vi "WinBuilder.vi"(6 "Wvfrm_ref":T1={"t0"=timestamp(0 s since 1904-01-01), "dt"=1.0, "attributes"=variant, "Y_ref"=refnum} {"dt" format="%0.6f"; "t0" format="%<%X\n%x>T"}, 8 "error in (no error)":errorcluster, 9 "AnalysisTime":dbl, 10 "clAnalysisConfig":T3={"F0"=60, "SettlingTime"=7.0, "AnalysisCycles"=20.0, "SampleRate"=4800.0, "NumChannels"=6, "TsOffset"=enum."start"}, 11 "Window":T2 {"T0" format="%.6f"; "Timestamp" format="%.6f"}) -> (0 "error out":errorcluster, 1 "Continue":bool, 2 "Valid":bool, 3 "Window":T2 {"T0" format="%.6f"; "Timestamp" format="%.6f"}, 4 "Wvfrm_ref":T1={"t0"=timestamp(0 s since 1904-01-01), "dt"=1.0, "attributes"=variant, "Y_ref"=refnum} {"dt" format="%0.6f"; "t0" format="%<%X\n%x>T"})   [LabVIEW 2018, in "AnalysisPlugins.lvlib" / "FitterBase.lvclass"]
uses:
  FitterBase.lvclass
  AnalysisPluginBaseClass/Typedefs/clWindowData.ctl
  Typedefs/clAnalysisConfig.ctl
  Typedefs/Wvfrm_ref.ctl
  Digitizer/DigitizerPlugins/DigitizerBaseClass/Typedefs/WfrmAttributes.ctl
  Digitizer/DigitizerPlugins/DigitizerBaseClass/DigitizerBase.lvclass
  AnalysisPluginBaseClass/AnalysisPluginsBase.lvclass
panel:
  out "AnalysisTime":timestamp
  out "SampleStartTime":timestamp
  out "TimestampNeeded":timestamp
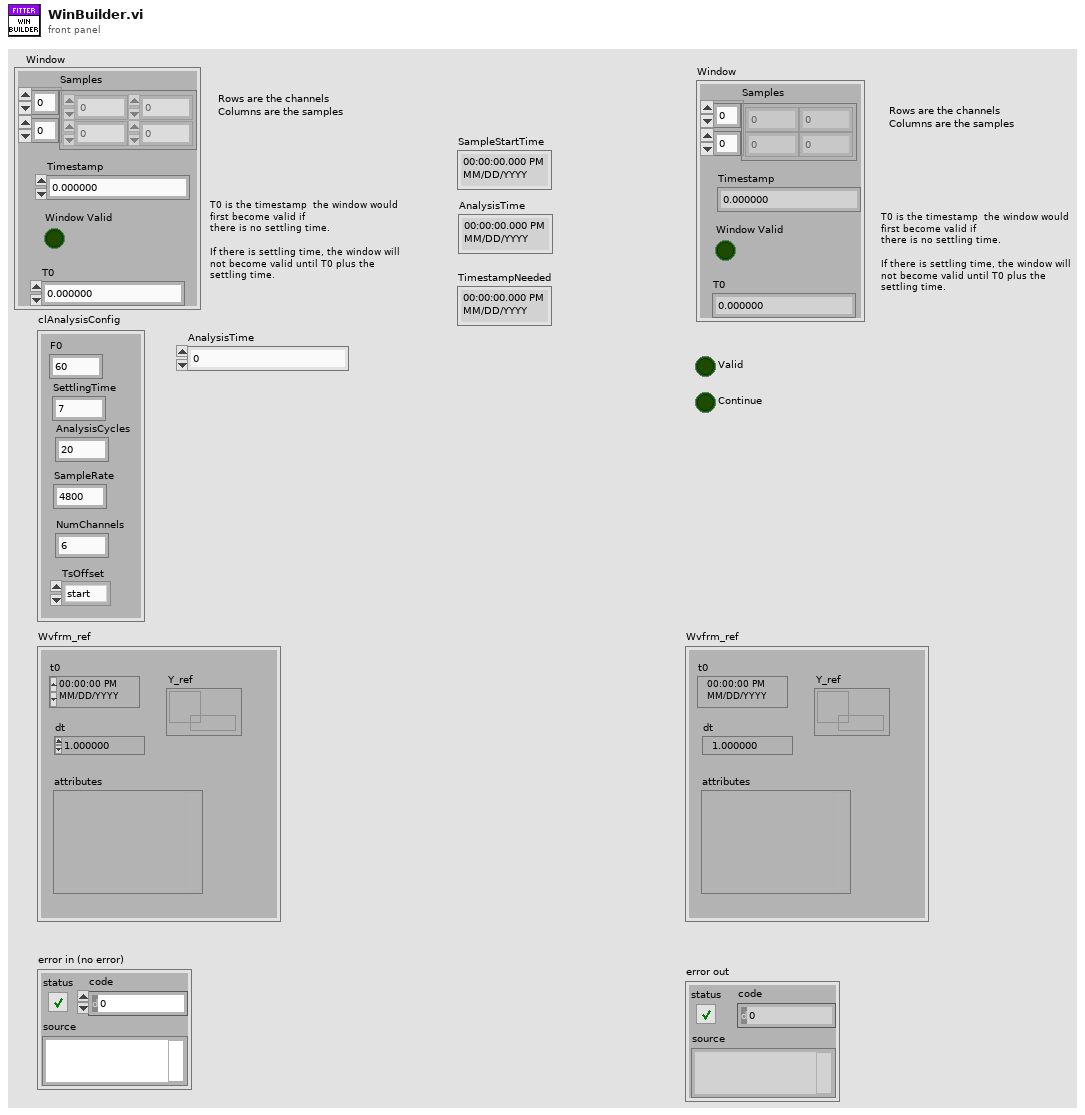
[diagram p1: front panel]
types:
  T1 = typedef "AnalysisPlugins.lvlib/FitterBase.lvclass/Wvfrm_ref.ctl" = cluster{"t0":timestamp, "dt":dbl, "attributes":variant, "Y_ref":refnum<data-value>}
  T2 = typedef "AnalysisPlugins.lvlib/AnalysisPluginsBase.lvclass/clWindowData.ctl" = cluster{"Timestamp":ext, "Samples":dbl[][], "Window Valid":bool, "T0":ext}
  T3 = typedef "AnalysisPlugins.lvlib/FitterBase.lvclass/clAnalysisConfig.ctl" = cluster{"F0":u32, "SettlingTime":dbl, "AnalysisCycles":dbl, "SampleRate":dbl, "NumChannels":u32, "TsOffset":enum16{"start", "middle", "end"}}
  T4 = typedef "DigitizerPlugins.lvlib/DigitizerBase.lvclass/WfrmAttributes.ctl" = cluster{"XOffset":dbl, "ActualPts":i64, "FirstValid":i64}
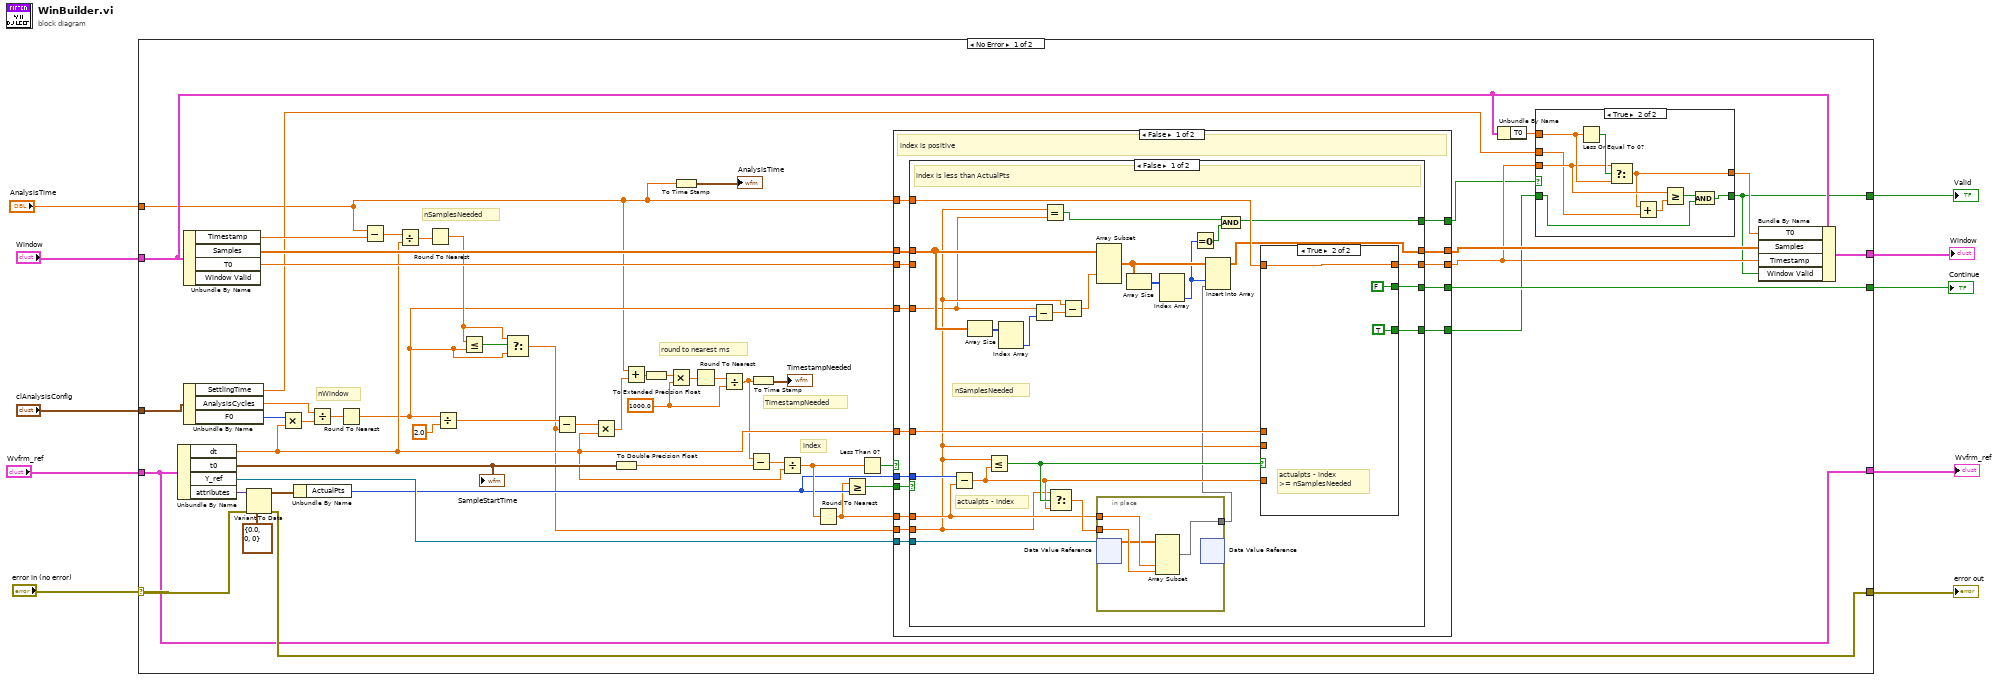
[diagram p0: block diagram]
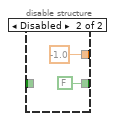
[diagram p3: hidden frame]
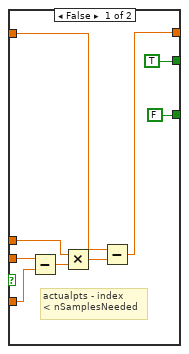
[diagram p4: hidden frame]
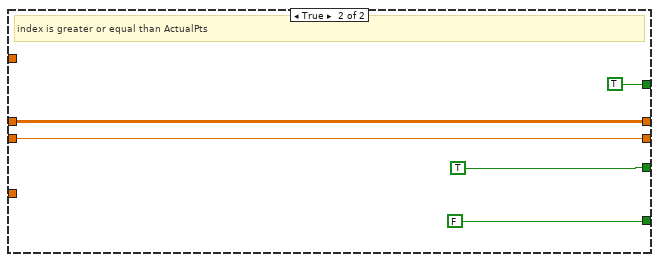
[diagram p5: hidden frame]
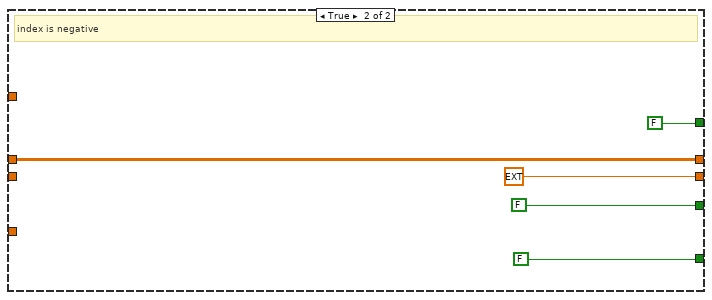
[diagram p6: hidden frame]
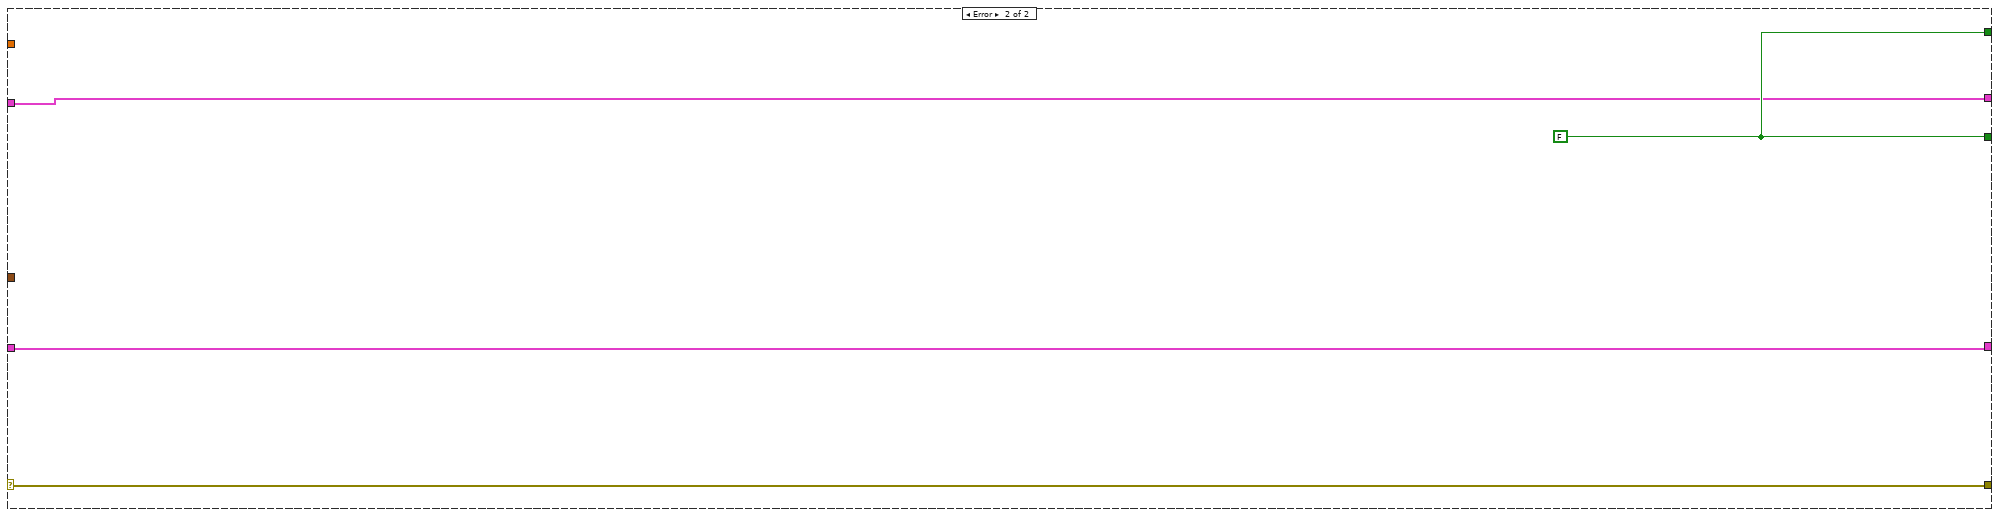
[diagram p7: hidden frame]
diagram:
  n1 = case shown="No Error" "error in (no error)" {
    selector: "error in (no error)" -> [w49 w152]
    tunnel: [w35 w152] -> w9
    tunnel: "AnalysisTime" -> [w18 _]
    tunnel: "Window" -> [w32 w150]
    tunnel: "Wvfrm_ref" -> [w21 w149]
    tunnel: "clAnalysisConfig" -> [w63 _]
    tunnel: [w40 w151] -> w4
    tunnel: [w26 w151] -> w3
    tunnel: [w33 w150] -> w2
    tunnel: [w21 w149] -> w1
    frame No Error {
      w14 = 1000.0
      # "round to nearest ms"
      # "index"
      # "TimestampNeeded"
      # "nWindow"
      # "nSamplesNeeded"
      n2 = Unbundle By Name(w21) -> ("dt"=w36:dbl, "t0"=w47:timestamp, "Y_ref"=w39:refnum<data-value>, "attributes"=w45:variant)
      "SampleStartTime" <- w47
      n3 = Unbundle By Name(w32) -> ("Timestamp"=w64:ext, "Samples"=w43:dbl[][], "T0"=w42:ext)  [unwired: 1 out]
      n4 = Unbundle By Name(w63) -> ("SettlingTime"=w31:dbl, "AnalysisCycles"=w60:dbl, "F0"=w62:u32)
      n5 = Variant To Data(error in=w49, type=T4 {"XOffset"=0.0, "ActualPts"=0, "FirstValid"=0} ("Attributes"), Variant=w45) -> (data=w50:T4, error out=w35:errorcluster)
      n6 = Multiply(x=w62, y=w36) -> (x*y=w61:dbl)
      n7 = Unbundle By Name(w50) -> ("ActualPts"=w37:i64)
      n8 = Divide(x=w60, y=w61) -> (x/y=w57:dbl)
      n9 = Round To Nearest(number=w57) -> (nearest integer value=w23:dbl)
      n10 = Subtract(x=w18, y=w64) -> (x-y=w59:ext)
      n11 = Divide(x=w59, y=w36) -> (x/y=w58:ext)
      n12 = Round To Nearest(number=w58) -> (nearest integer value=w24:ext)
      n13 = Divide(x=w23, y=2.0) -> (x/y=w55:dbl)
      n14 = Less Or Equal?(x=w24, y=w23) -> (x <= y?=w25:bool)
      n15 = Select(t=w24, s=w25, f=w23) -> (s? t:f=w22:ext)
      n16 = Subtract(x=w55, y=w22) -> (x-y=w54:ext)
      n17 = Multiply(x=w54, y=w36) -> (x*y=w53:ext)
      n18 = To Double Precision Float(number=w47) -> (double precision float=w48:dbl)
      n19 = Add(x=w18, y=w53) -> (x+y=w12:ext)
      n20 = To Extended Precision Float(1:w12) -> (0:w11:ext)
      n21 = Multiply(x=w11, y=w14) -> (x*y=w16:ext)
      n22 = To Time Stamp(1:w18) -> (0:→"AnalysisTime":timestamp)
      n23 = Round To Nearest(number=w16) -> (nearest integer value=w15:ext)
      n24 = Divide(x=w15, y=w14) -> (x/y=w13:ext)
      n25 = Subtract(x=w13, y=w48) -> (x-y=w46:ext)
      n26 = To Time Stamp(1:w13) -> (0:→"TimestampNeeded":timestamp)
      n27 = Divide(x=w46, y=w36) -> (x/y=w38:ext)
      n28 = Round To Nearest(number=w38) -> (nearest integer value=w19:ext)
      n29 = Greater Or Equal?(x=w19, y=w37) -> (x >= y?=w41:bool)
      n30 = Less Than 0?(x=w38) -> (x < 0?=w44:bool)
      n31 = case shown="False" w44 {
        tunnel: w43 -> [w95 w148]
        tunnel: [w94 w148] -> w34
        tunnel: w42 -> [w93 _]
        tunnel: w41 -> [w96 _]
        tunnel: [w92 ext 0.0 ("T0")] -> w28
        tunnel: [w91 FALSE] -> w40
        tunnel: w39 -> [w90 _]
        tunnel: w19 -> [w89 _]
        tunnel: w22 -> [w88 _]
        tunnel: w23 -> [w87 _]
        tunnel: w18 -> [w86 _]
        tunnel: w37 -> [w85 _]
        tunnel: w36 -> [w84 _]
        tunnel: [w83 FALSE] -> w29
        tunnel: [w82 FALSE] -> w20
        frame False {
          # "index is positive"
          n32 = case shown="False" w96 {
            tunnel: w95 -> [w121 w143]
            tunnel: [w102 w143] -> w94
            tunnel: w93 -> [_ w142]
            tunnel: [w115 w142] -> w92
            tunnel: [w118 TRUE] -> w91
            tunnel: w90 -> [w108 _]
            tunnel: w89 -> [w106 _]
            tunnel: w88 -> [w101 _]
            tunnel: w87 -> [w100 _]
            tunnel: w86 -> [w116 _]
            tunnel: w85 -> [w117 _]
            tunnel: w84 -> [w114 _]
            tunnel: [w113 FALSE] -> w83
            tunnel: [w98 TRUE] -> w82
            frame False {
              # "nSamplesNeeded"
              # "actualpts - index"
              # "index is less than ActualPts"
              n33 = Subtract(x=w117, y=w106) -> (x-y=w109:ext)
              n34 = Array Size(array=w121) -> (size(s)=w122:i32[])
              n35 = Less Or Equal?(x=w101, y=w109) -> (x <= y?=w110:bool)
              n36 = Index Array(array=w122) -> (element #2=w112:i32)  [unwired: 2 in, 1 out]
              n37 = Subtract(x=w100, y=w112) -> (x-y=w120:dbl)
              n38 = Equal?(x=w101, y=w100) -> (x = y?=w99:bool)
              n39 = Select(t=w101, s=w110, f=w109) -> (s? t:f=w107:ext)
              n40 = Subtract(x=w101, y=w120) -> (x-y=w119:ext)
              n41 = Array Subset(array=w121, index (col)=w119) -> (w105:dbl[][])  [unwired: 3 in]
              n42 = in-place {
                in-place-border: w106 -> [w124]
                in-place-border: w107 -> [w125]
                in-place-border: [w126] -> w103
                n43 = in-place-dvr #1(w108) -> (w123:dbl[][])  [unwired: 1 out]
                n44 = Array Subset(array=w123, index (col)=w124, length (col)=w125) -> (w126:dbl[][])  [unwired: 2 in]
                n45 = in-place-dvr #1() -> ()  [unwired: 1 in, 2 out]
              }
              n46 = Array Size(array=w105) -> (size(s)=w111:i32[])
              n47 = Index Array(array=w111) -> (element #2=w104:i32)  [unwired: 2 in, 1 out]
              n48 = Equal To 0?(x=w104) -> (x = 0?=w97:bool)
              n49 = Insert Into Array(array=w105, index (col)=w104, new element=w103) -> (w102:dbl[][])  [unwired: 1 in]
              n50 = And(x=w99, y=w97) -> (x .and. y?=w98:bool)
              n51 = case shown="True" w110 {
                tunnel: [TRUE FALSE] -> w118
                tunnel: w116 -> [w130 w137]
                tunnel: [w129 w137] -> w115
                tunnel: w109 -> [w127 _]
                tunnel: w101 -> [w134 _]
                tunnel: w114 -> [w132 _]
                tunnel: [FALSE TRUE] -> w113
                frame False {
                  # "actualpts - index\n< nSamplesNeeded"
                  n52 = Subtract(x=w134, y=w127) -> (x-y=w133:ext)
                  n53 = Multiply(x=w132, y=w133) -> (x*y=w131:ext)
                  n54 = Subtract(x=w130, y=w131) -> (x-y=w129:ext)
                }
                frame True {
                  # "actualpts - index\n>= nSamplesNeeded"
                }
              }
            }
            frame True {
              # "index is greater or equal than ActualPts"
            }
          }
        }
        frame True {
          # "index is negative"
        }
      }
      n55 = Unbundle By Name(w32) -> ("T0"=w30:ext)
      n56 = case shown="True" w20 {
        tunnel: w30 -> [w65 w80]
        tunnel: w31 -> [_ w76]
        tunnel: w28 -> [_ w79]
        tunnel: [w66 w77] -> w27
        tunnel: [w67 w75] -> w26
        tunnel: w29 -> [w68 w73]
        frame False {
          n57 = disable-structure shown="Enabled" {
            disable-tunnel: w68 -> [w70 _]
            disable-tunnel: [w70 FALSE] -> w67
            disable-tunnel: [w69 -1.0] -> w66
            disable-tunnel: w65 -> [w69 _]
            frame Enabled {
            }
            frame Disabled {
            }
          }
        }
        frame True {
          n58 = Less Or Equal To 0?(x=w80) -> (x <= 0?=w81:bool)
          n59 = Select(t=w79, s=w81, f=w80) -> (s? t:f=w77:ext)
          n60 = Add(x=w77, y=w76) -> (x+y=w78:ext)
          n61 = Greater Or Equal?(x=w79, y=w78) -> (x >= y?=w74:bool)
          n62 = And(x=w74, y=w73) -> (x .and. y?=w75:bool)
        }
      }
      n63 = Bundle By Name(cluster=w32, "T0"=w27, "Samples"=w34, "Timestamp"=w28, "Window Valid"=w26) -> (w33:T2)
    }
    frame Error {
      w151 = FALSE
    }
  }
  "Window" <- w2
  "Wvfrm_ref" <- w1
  "Valid" <- w3
  "Continue" <- w4
  "error out" <- w9
